vi "Destroy.vi"(0 "reference in":refnum<class "BKP-891 LCR Meter.lvclass">, 5 "error in (no error)":errorcluster) -> (14 "reference out":refnum<class "BKP-891 LCR Meter.lvclass">, 19 "error out":errorcluster)   [LabVIEW 2018, in "BKP-891 LCR Meter.lvclass"]
uses:
  BKP-891 LCR Meter.lvclass
  <instrlib>/BK Precision 891/BK Precision 891.lvlib
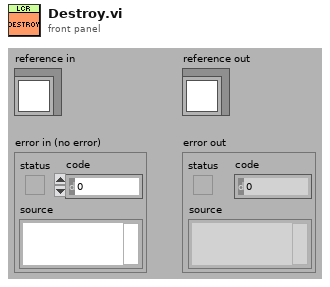
[diagram p1: front panel]
types:
  T1 = typedef "BKP-891 LCR Meter.lvclass/ObjectAttributes.ctl" = cluster{"VISA resource name":refnum<visa-resource-name>, "Simulated?":bool, "Latest Values":dbl[], "Signal List":T2[], "Tare Offset":dbl[], "Range":u16, "Measurement Speed":u16, "Function":u16, "Signal Frequency (Hz)":dbl, "Signal Level (Vrms)":u8, "UVW Mode":enum16{"UV", "UW", "VW"}, "LR Mode":T3, "Primary Parameter":string, "Secondary Parameter":string}
  T2 = typedef "IO Signal List.ctl" = enum16{"Timestamp", "PSU_FB_U_VDC", "PSU_FB_I_AMP", "PSU_FB_W_WATT", "PSU_CMD_U_VDC", "PSU_CMD_I_AMP", "PSU_CMD_OUTPUT", "LCR_PRIMARY", "LCR_SECONDARY", "UV_R_mOhm", "UW_R_mOhm", "VW_R_mOhm", "UV_L_µH", "UW_L_µH", "VW_L_µH", "U_U_VDC", "V_U_VDC", "W_U_VDC", "U_I_AMP", "V_I_AMP", "W_I_AMP", "PWM_CMD_DC_%", "PWM_CMD_VDC", "PWM_CMD_Hz", "PWM_FB_DC_%", "PWM_FB_VDC", "PWM_FB_Hz", "DO_RELAY_U_LCR_A", "DO_RELAY_V_LCR_A", "DO_RELAY_V_LCR_B", "DO_RELAY_W_LCR_B", "DIFF_UV_UW_L_µH", "DIFF_UV_VW_L_µH", "DIFF_UW_VW_L_µH", "DIFF_UV_UW_R_mOhm", "DIFF_UV_VW_R_mOhm", "DIFF_UW_VW_R_mOhm", "DIFF_UV_U_VDC", "DIFF_UW_U_VDC", "DIFF_VW_U_VDC"}
  T3 = typedef "LR Mode.ctl" = enum16{"R - Resistance", "L - Inductance"}
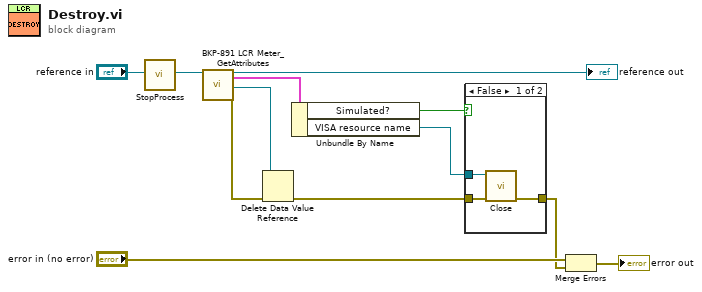
[diagram p0: block diagram]
diagram:
  n1 = call "StopProcess.vi"("reference in"="reference in") -> ("reference out"=w5:refnum<class "BKP-891 LCR Meter.lvclass">)  [unwired: 17 in, 1 out]
  n2 = call "BKP-891 LCR Meter_GetAttributes.vi"("reference in"=w5) -> ("reference out"=→"reference out":refnum<class "BKP-891 LCR Meter.lvclass">, "Data"=w8:T1, "DataRef"=w9:refnum<data-value>, "error out"=w10:errorcluster)  [unwired: 15 in]
  n3 = Delete Data Value Reference(data value reference=w9, error in=w10) -> (error out=w4:errorcluster)  [unwired: 1 out]
  n4 = Unbundle By Name(w8) -> ("Simulated?"=w1:bool, "VISA resource name"=w2:refnum<visa-resource-name>)
  n5 = case shown="False" w1 {
    tunnel: w4 -> [w15 w16]
    tunnel: [w14 w16] -> w3
    tunnel: w2 -> [w13 _]
    frame False {
      n6 = call <instrlib>:"Close.vi"("error in (no error)"=w15, "VISA resource name"=w13) -> ("error out"=w14:errorcluster)  [unwired: 9 in]
    }
    frame True {
    }
  }
  n7 = Merge Errors("error in (no error)", w3) -> (→"error out":errorcluster)
